vi "Test Remove Quotes from String if Present.vi"(8 "error in (no error)":errorcluster) -> (0 "error out":errorcluster)   [LabVIEW 2013, in "TEST JKI State Machine API.lvlib"]
uses:
  TEST JKI State Machine API.lvlib
  <vilib>/addons/_JKI Toolkits/Caraya/classes/Assert/Assert.lvclass
  <vilib>/addons/_JKI Toolkits/Caraya/classes/Test/Test.lvclass
  source/JKI SM/JKI SM.lvclass
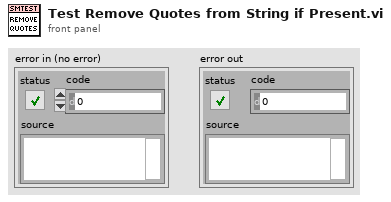
[diagram p1: front panel]
types:
  T1 = cluster{"Input":string, "Expected Output":string, "Comment":string}[]
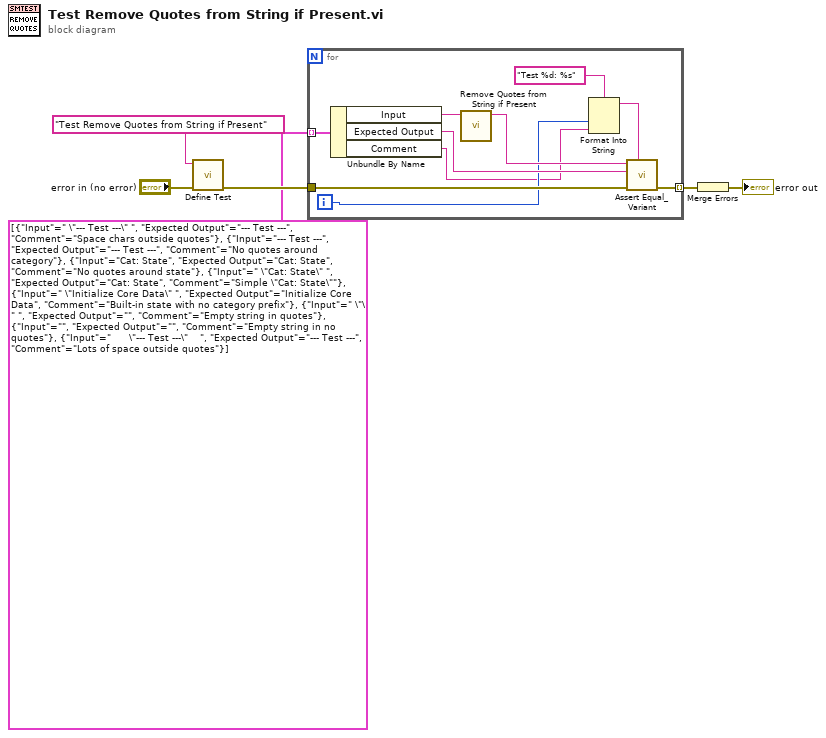
[diagram p0: block diagram]
diagram:
  n1 = call <vilib>:"Define Test.vi"("error in (no error)"="error in (no error)", "Label (VI Title)"="Test Remove Quotes from String if Present") -> ("error out"=w3:errorcluster)  [unwired: 9 in]
  n2 = for {
    tunnel: [w16] -> w4 mode=indexing
    tunnel: w3 -> [w15]
    tunnel: T1 [{"Input"=" \"--- Test ---\" ", "Expected Output"="--- Test ---", "Comment"="Space chars outside quotes"}, {"Input"="--- Test ---", "Expected Output"="--- Test ---", "Comment"="No quotes around category"}, {"Input"="Cat: State", "Expected Output"="Cat: State", "Comment"="No quotes around state"}, {"Input"=" \"Cat: State\" ", "Expected Output"="Cat: State", "Comment"="Simple \"Cat: State\""}, {"Input"=" \"Initialize Core Data\" ", "Expected Output"="Initialize Core Data", "Comment"="Built-in state with no category prefix"}, {"Input"=" \"\" ", "Expected Output"="", "Comment"="Empty string in quotes"}, {"Input"="", "Expected Output"="", "Comment"="Empty string in no quotes"}, {"Input"="      \"--- Test ---\"    ", "Expected Output"="--- Test ---", "Comment"="Lots of space outside quotes"}] -> [w14] mode=indexing
    i -> [w9]
    n3 = Unbundle By Name(w14) -> ("Input"=w10:string, "Expected Output"=w11:string, "Comment"=w8:string)
    n4 = call "Remove Quotes from String if Present.vi"("String"=w10) -> ("String with Quotes Removed"=w13:string)  [unwired: 10 in]
    n5 = Format Into String(format string="Test %d: %s", w9, w8) -> (resulting string=w7:string)  [unwired: 2 in, 1 out]
    n6 = call <vilib>:"Assert Equal_Variant.vi"("Label"=w7, "error in (no error)"=w15, "Y"=w11, "X"=w13) -> ("error out"=w16:errorcluster)  [unwired: 7 in]
  }
  n7 = Merge Errors(w4) -> (→"error out":errorcluster)
